vi "Create Channel.vi"(8 "error in (no error)":errorcluster, 10 "I/O":T1, 11 "National Instrument USB-6501 in":refnum<class "National Instrument USB-6501.lvclass">) -> (0 "error out":errorcluster, 1 "Channel out":refnum<k21>, 2 "Cluster":T2, 3 "National Instrument USB-6501 out":refnum<class "National Instrument USB-6501.lvclass">)   [LabVIEW 2016, in "Generic Data Acquisition.lvlib" / "National Instrument USB-6501.lvlib" / "National Instrument USB-6501.lvclass"]
uses:
  National Instrument USB-6501.lvclass
  Controls/Data Acquisition Channel Settings.ctl
  <vilib>/DAQmx/create/channels.llb/DAQmx Create Channel (DI-Digital Input).vi
  <vilib>/DAQmx/create/channels.llb/DAQmx Create Channel (DO-Digital Output).vi
  <resource>/objmgr/daqmx.rc
panel:
  out "IsGlobal":bool
  out "task out":refnum<k21>
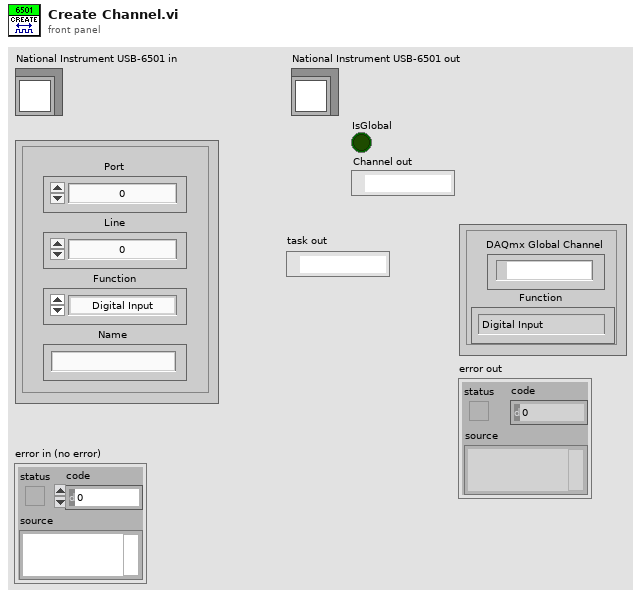
[diagram p1: front panel]
types:
  T1 = typedef "Data Acquisition Channel Settings.ctl" = cluster{"Function":enum16{"Digital Input", "Digital Output"}, "Port":i8, "Line":i8, "Name":string}
  T2 = cluster{"Function":enum16{"Digital Input", "Digital Output"}, "DAQmx Global Channel":refnum<k21>}
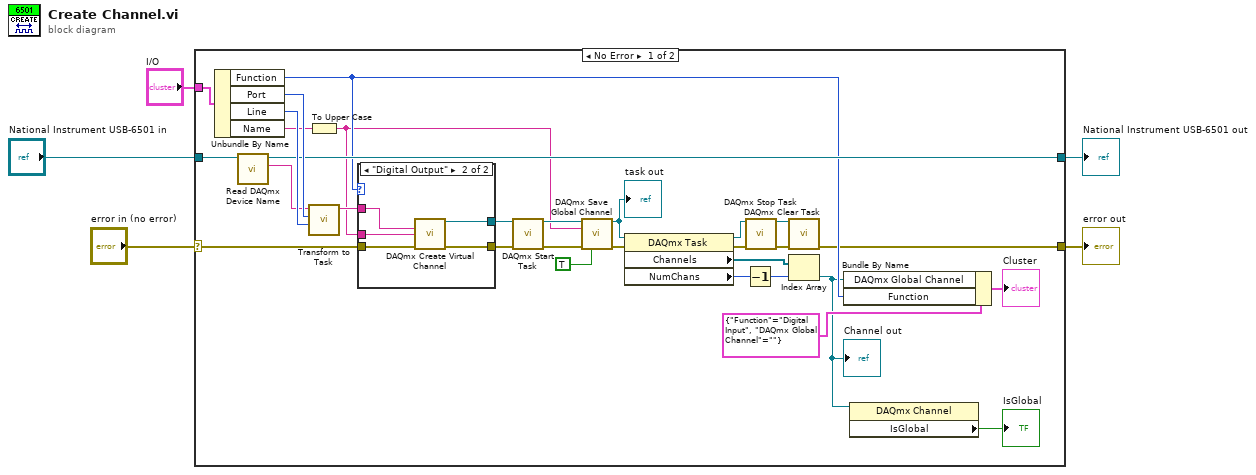
[diagram p0: block diagram]
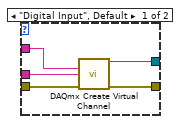
[diagram p2: hidden frame]
diagram:
  n1 = case shown="No Error" "error in (no error)" {
    selector: "error in (no error)" -> [w32 w47]
    tunnel: [w7 w47] -> w4
    tunnel: [w28 w46] -> w2
    tunnel: "National Instrument USB-6501 in" -> [w30 w46]
    tunnel: "I/O" -> [w35 _]
    frame No Error {
      n2 = Unbundle By Name(w35) -> ("Function"=w27:enum16{"Digital Input", "Digital Output"}, "Port"=w34:i8, "Line"=w33:i8, "Name"=w6:string)
      n3 = call-dynamic "Read DAQmx Device Name.vi"("National Instrument USB-6501 in"=w30) -> ("DAQmx Device Name"=w29:tag, "National Instrument USB-6501 out"=w28:refnum<class "National Instrument USB-6501.lvclass">)  [unwired: 8 in, 1 out]
      n4 = To Upper Case(1:w6) -> (0:w16:string)
      n5 = call "Transform to Task.vi"("Line"=w33, "Port"=w34, "DAQmx Device Name"=w29) -> ("Classic DAQmx Physical Channel"=w23:tag)  [unwired: 8 in]
      n6 = case shown="\"Digital Output\"" w27 {
        tunnel: w32 -> [w38 w45]
        tunnel: [w37 w44] -> w31
        tunnel: [w36 w43] -> w24
        tunnel: w23 -> [w40 w42]
        tunnel: w16 -> [w39 w41]
        frame "Digital Input", Default {
          n7 = call-poly <vilib>:"DAQmx Create Virtual Channel.vi"("lines"=w40, "name to assign"=w39, "error in"=w38) -> ("task out"=w36:refnum<k21>, "error out"=w37:errorcluster)  [unwired: 11 in]
        }
        frame "Digital Output" {
          n8 = call-poly <vilib>:"DAQmx Create Virtual Channel.vi"("lines"=w42, "name to assign"=w41, "error in"=w45) -> ("task out"=w43:refnum<k21>, "error out"=w44:errorcluster)  [unwired: 11 in]
        }
      }
      n9 = call <vilib>:"DAQmx Start Task.vi"("task/channels in"=w24, "error in"=w31) -> ("task out"=w25:refnum<k21>, "error out"=w26:errorcluster)  [unwired: 12 in]
      n10 = call <vilib>:"DAQmx Save Global Channel.vi"("task/channels in"=w25, "channel name"=w16, "error in"=w26, "overwrite existing channel?"=TRUE) -> ("task out"=w22:refnum<k21>, "error out"=w8:errorcluster)  [unwired: 10 in]
      "task out" <- w22
      n11 = property class="DAQmx Task"(reference=w22, error in=w8) -> (reference out=w12:refnum<k21>, error out=w9:errorcluster, "Channels"=w21:refnum<k21>[], "NumChans"=w20:u32)
      n12 = Decrement(x=w20) -> (x-1=w19:u32)
      n13 = call <vilib>:"DAQmx Stop Task.vi"("task/channels in"=w12, "error in"=w9) -> ("task out"=w11:refnum<k21>, "error out"=w10:errorcluster)  [unwired: 12 in]
      n14 = call <vilib>:"DAQmx Clear Task.vi"("task in"=w11, "error in"=w10) -> ("error out"=w7:errorcluster)  [unwired: 13 in]
      n15 = Index Array(array=w21, index=w19) -> (element=w13:refnum<k21>)
      "Channel out" <- w13
      n16 = Bundle By Name(cluster=T2 {"Function"=enum."Digital Input", "DAQmx Global Channel"=""} ("Cluster"), "DAQmx Global Channel"=w13, "Function"=w27) -> (→"Cluster":T2)
      n17 = property class="DAQmx Channel"(reference=w13) -> ("IsGlobal"=→"IsGlobal":bool)  [unwired: 1 in, 2 out]
    }
    frame Error {
    }
  }
  "error out" <- w4
  "National Instrument USB-6501 out" <- w2
